vi "Romi-Robot-Simulation.vi"() -> ()   [LabVIEW 2019]
doc: "This WebSockets API example VI acts as a server for an incoming websockets connection. Receives/sends string data to the connected client."
uses:
  <vilib>/Rock Robotics/WPI/Simulation/Protocol/Devices/RoboRIO/RoboRIO Update Ops.ctl
  <vilib>/Rock Robotics/WPI/Simulation/Protocol/Devices/DriverStation/DS Update Ops.ctl
  <vilib>/Rock Robotics/WPI/Simulation/Protocol/Devices/DIO/DIO Update Ops.ctl
  <vilib>/Rock Robotics/SystemInterfaces/DIO/FPGA_DIOChannel.ctl
  <vilib>/Utility/miscctls.llb/LVBoundsTypeDef.ctl
  <vilib>/Rock Robotics/WPI/ThirdParty/JAS_Junk/TrajLib/Trajectory_Library.lvlib
  <vilib>/mediamongrels ltd/websockets/websockets/websocket server/WebSocket Server.lvclass
  C:/Program Files (x86)/National Instruments/LabVIEW 2020/vi.lib/mediamongrels ltd/websockets/websockets/websocket/WebSocket.lvclass
  <vilib>/Rock Robotics/WPI/Simulation/Protocol/Devices/PWM/PWM data proto.ctl
  <vilib>/Rock Robotics/WPI/Simulation/Protocol/Devices/PWM/PWM proto.ctl
  <vilib>/Rock Robotics/WPI/Simulation/Protocol/Devices/RoboRIO/RoboRIO data proto.ctl
  <vilib>/Rock Robotics/WPI/Simulation/Protocol/Devices/RoboRIO/RoboRIO proto.ctl
  <vilib>/Rock Robotics/WPI/Simulation/Protocol/Devices/DriverStation/DS data proto.ctl
  <vilib>/Rock Robotics/WPI/Simulation/Protocol/Devices/DriverStation/DS proto.ctl
  <vilib>/Rock Robotics/WPI/Simulation/Protocol/Devices/DIO/DIO data proto.ctl
  <vilib>/Rock Robotics/WPI/Simulation/Protocol/Devices/DIO/DIO proto.ctl
  <vilib>/Rock Robotics/WPI/Simulation/Protocol/Devices/Encoder/Encoder data protoo.ctl
  <vilib>/Rock Robotics/WPI/Simulation/Protocol/Devices/Encoder/Encoder proto.ctl
  <vilib>/Analysis/Matrix/Datatypes/RealMatrix.ctl
  <vilib>/Analysis/Matrix/NI_Matrix.lvlib
  <vilib>/Rock Robotics/WPI/ThirdParty/JAS_Junk/TrajLib/TypeDef/LINEAR_SYSTEM.ctl
  <vilib>/Rock Robotics/WPI/ThirdParty/JAS_Junk/TrajLib/TypeDef/DCMOTOR.CTL
  <vilib>/Rock Robotics/WPI/ThirdParty/JAS_Junk/TrajLib/TypeDef/DIFF_DRIVE_TRAIN_SIM.ctl
  <vilib>/vision/Image Controls.llb/IMAQ Image.ctl
  ROBOT_PICTURE.ctl
  <vilib>/Rock Robotics/WPI/Simulation/Protocol/Devices/Gyro/Gyro Data proto.ctl
  <vilib>/Rock Robotics/WPI/Simulation/Protocol/Devices/Gyro/Gyro proto.ctl
panel:
  in  "Tab Control":T1(tab)
  in  "Start Simulation":bool
  in  "Field Selector":string(combo)
  in  "Robot Y Position\nInches":dbl=84.0
  in  "Robot X Position\nInches":dbl=120.0
  in  "Robot Orientation\nDegrees":dbl
  out "Heading Deg":dbl format="%11.1f"
  out "Right Wheel\nInch / Sec":dbl format="%11.1f"
  out "Left Wheel\nInch / Sec":dbl format="%11.1f"
  in  "Button\n    C":bool
  in  "Button\n    B":bool
  out "Yellow LED\nDIO 3":bool
  out "Green LED\nDIO 1":bool
  out "Red LED\nDIO 2":bool
  in  "Button\n    A":bool
  out "RSL ON":picture
  out "ROBOT":T2
  out "RSL OFF":picture
  out "Field Picture":picture
  out "Y Pos Inch":dbl format="%11.1f"
  out "X Pos Inch":dbl format="%11.1f"
  out "Gyro":T3={"type"="Gyro", "device"="", "name"="", "data"={"<init"=0, ">connected"=FALSE, "<offsetX"=0.0, "<offsetY"=0.0, "<offsetZ"=0.0, ">angle_x"=0.0, ">angle_y"=0.0, ">angle_z"=0.0, ">rate_x"=0.0, ">rate_y"=0.0, ">rate_z"=0.0, "<gain"=0.0}}
  out "DIO 0\nIn":T5={"type"="DIO", "device"="", "name"="", "data"={"<init"=FALSE, "<>value"=FALSE, "<pulse_length"=0, "<input"=FALSE}}
  out "Enc Left":T7={"type"="Encoder", "device"="", "name"="", "data"={"<init"=FALSE, ">count"=0.0, ">period"=0.0, "<samples_to_avg"=0, "<offset"=0.0, "<channel_a"=0, "<channel_b"=0}}
  out "Enc Right":T7={"type"="Encoder", "device"="", "name"="", "data"={"<init"=FALSE, ">count"=0.0, ">period"=0.0, "<samples_to_avg"=0, "<offset"=0.0, "<channel_a"=0, "<channel_b"=0}}
  out "DIO 1\nIn / Out":T5={"type"="DIO", "device"="", "name"="", "data"={"<init"=FALSE, "<>value"=FALSE, "<pulse_length"=0, "<input"=FALSE}}
  out "DIO 2\nIn / Out":T5={"type"="DIO", "device"="", "name"="", "data"={"<init"=FALSE, "<>value"=FALSE, "<pulse_length"=0, "<input"=FALSE}}
  out "PWM 0":T9
  out "PWM 1":T9
  out "DIO 3\nOut":T5={"type"="DIO", "device"="", "name"="", "data"={"<init"=FALSE, "<>value"=FALSE, "<pulse_length"=0, "<input"=FALSE}}
  out "roboRIO":T11={"type"="roboRIO", "device"="", "name"="", "data"={">fpga_button"=FALSE, ">vin_voltage"=0.0, ">vin_current"=0.0, ">6v_voltage"=0.0, ">6v_current"=0.0, ">6v_active"=FALSE, ">6v_faults"=0.0, ">5v_voltage"=0.0, ">5v_current"=0.0, ">5v_active"=FALSE, ">5v_faults"=0.0, ">3v3_voltage"=0.0, ">3v3_current"=0.0, ">3v3_active"=FALSE, ">3v3_faults"=0.0}}
  out "Driverstation":T13={"type"="Driverstation", "device"="", "name"="", "data"={">enabled"=FALSE, ">autonomous"=FALSE, ">test"=FALSE, ">estop"=FALSE, ">fms"=FALSE, ">ds"=FALSE, "<match_time"=0.0, ">station"="", ">game_data"=""}}
  out "Request URI":string
  out "HTTP Headers":variant
  out "Stop Sim":bool
  out "Battery Voltage VDC":dbl format="%18.2f"
  out "Gyro Reading   Deg":dbl format="%19.3f"
  out "Edges/Feet":dbl
  out "out DiffDriveTrainSim":T15 {"m_Motor"."Jr_KgM2" format="%13.5p"; "m_Motor"."L_H" format="%13.5p"; "m_Motor"."Kt_NMPerAmp" format="%13.5p"; "m_Motor"."KvINV_RadPerSecPerVolt" format="%13.5p"; "m_Motor"."R_Ohms" format="%13.5p"; "m_Motor"."FreeSpeed_RadPerSec" format="%13.5p"; "m_Motor"."FreeCurrent_Amps" format="%13.5p"; "m_Motor"."StallCurrent_Amps" format="%13.5p"; "m_Motor"."StallTorque_NM" format="%13.5p"; "m_Motor"."nominalVoltage_Volts" format="%13.5p"}
  out "Speed Left  Ft/Sec":dbl format="%13.2f"
  out "Speed Right  Ft/Sec":dbl format="%13.2f"
  out "Amps":dbl
  out "PWM 0 Rate":dbl format="%19.3f"
  out "PWM 1 Rate":dbl format="%19.3f"
  out "FIeld Image":T19
  out "Y Pos Pixel":dbl format="%11.1f"
  out "X Pos Pixel":dbl format="%11.1f"
  # "Romi Switches/Lights"
  # "Robot Position"
  # "Robot Speed"
  # "Dig In 0"
  # "Dig In 1"
  # "Dig In 2"
  # "<States, 1>"
  # "<Outputs, 1>"
  # "<Inputs, 1>"
  # "<Outputs, 1>"
  # "<States,States>"
  # "<States,Inputs>"
  # "<Outputs,States>"
  # "<Outputs,Inputs>"
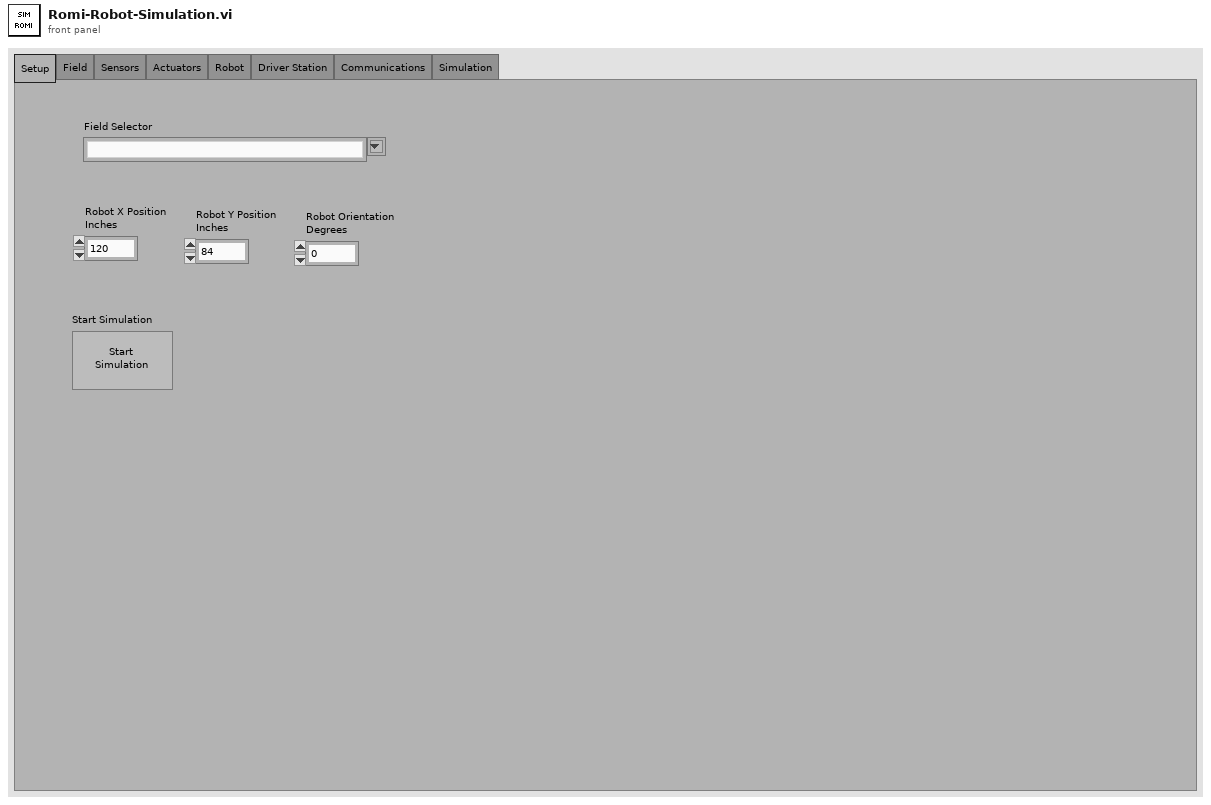
[diagram p1: front panel]
types:
  T1 = enum32{"Setup", "Field", "Sensors", "Actuators", "Robot", "Driver Station", "Communications", "Simulation"}
  T2 = typedef "ROBOT_PICTURE.ctl" = picture
  T3 = typedef "Gyro proto.ctl" = cluster{"type":string, "device":string, "name":string, "data":T4}
  T4 = typedef "Gyro Data proto.ctl" = cluster{"<init":i32, ">connected":bool, "<offsetX":dbl, "<offsetY":dbl, "<offsetZ":dbl, ">angle_x":dbl, ">angle_y":dbl, ">angle_z":dbl, ">rate_x":dbl, ">rate_y":dbl, ">rate_z":dbl, "<gain":dbl}
  T5 = typedef "DIO proto.ctl" = cluster{"type":string, "device":string, "name":string, "data":T6}
  T6 = typedef "DIO data proto.ctl" = cluster{"<init":bool, "<>value":bool, "<pulse_length":i32, "<input":bool}
  T7 = typedef "Encoder proto.ctl" = cluster{"type":string, "device":string, "name":string, "data":T8}
  T8 = typedef "Encoder data protoo.ctl" = cluster{"<init":bool, ">count":dbl, ">period":dbl, "<samples_to_avg":i32, "<offset":dbl, "<channel_a":i32, "<channel_b":i32}
  T9 = typedef "PWM proto.ctl" = cluster{"type":string, "device":string, "name":string, "data":T10}
  T10 = typedef "PWM data proto.ctl" = cluster{"<init":bool, "<speed":dbl, "<position":dbl, "<raw":dbl, "<period_scale":dbl, "<zero_latch":bool, "<servo range":dbl}
  T11 = typedef "RoboRIO proto.ctl" = cluster{"type":string, "device":string, "name":string, "data":T12}
  T12 = typedef "RoboRIO data proto.ctl" = cluster{">fpga_button":bool, ">vin_voltage":dbl, ">vin_current":dbl, ">6v_voltage":dbl, ">6v_current":dbl, ">6v_active":bool, ">6v_faults":dbl, ">5v_voltage":dbl, ">5v_current":dbl, ">5v_active":bool, ">5v_faults":dbl, ">3v3_voltage":dbl, ">3v3_current":dbl, ">3v3_active":bool, ">3v3_faults":dbl}
  T13 = typedef "DS proto.ctl" = cluster{"type":string, "device":string, "name":string, "data":T14}
  T14 = typedef "DS data proto.ctl" = cluster{">enabled":bool, ">autonomous":bool, ">test":bool, ">estop":bool, ">fms":bool, ">ds":bool, "<match_time":dbl, ">station":string, ">game_data":string}
  T15 = typedef "Trajectory_Library.lvlib/DIFF_DRIVE_TRAIN_SIM.ctl" = cluster{"m_Plant":T16, "m_X":T17, "m_Y":T17, "m_U":T17, "MeasureStdDev":T17, "m_Motor":T18, "m_OriginalGearing":dbl, "m_CurrentGearing":dbl, "m_WheelRadius_M":dbl, "m_RB":dbl}
  T16 = typedef "Trajectory_Library.lvlib/LINEAR_SYSTEM.ctl" = cluster{"m_A":T17, "m_B":T17, "m_C":T17, "m_D":T17, "States":i32, "Inputs":i32, "Outputs":i32}
  T17 = typedef "NI_Matrix.lvlib/RealMatrix.ctl" = dbl[][]
  T18 = typedef "Trajectory_Library.lvlib/DCMOTOR.CTL" = cluster{"nominalVoltage_Volts":dbl, "StallTorque_NM":dbl, "StallCurrent_Amps":dbl, "FreeCurrent_Amps":dbl, "FreeSpeed_RadPerSec":dbl, "R_Ohms":dbl, "KvINV_RadPerSecPerVolt":dbl, "Kt_NMPerAmp":dbl, "L_H":dbl, "Jr_KgM2":dbl}
  T19 = typedef "IMAQ Image.ctl" = refnum<image>
  T20 = typedef "LVBoundsTypeDef.ctl" = cluster{"Width":u32, "Height":u32}
  T21 = typedef "Image Type" = u32
  T22 = typedef "TrajectoryUtils_Field_Info.ctl" = cluster{"FIeld_File_Name":string, "Top_Left_X":i32, "Top_Left_Y":i32, "Bottom_Right_X":i32, "Bottom_Right_Y":i32, "Field_Size_X":dbl, "Field_Size_Y":dbl, "FIeld_Size_Units":string}
  T23 = typedef "Trajectory_Library.lvlib/POSE2D.ctl" = cluster{"TRANSLATION":T24, "ROTATION":T25}
  T24 = typedef "Trajectory_Library.lvlib/TRANSLATION2D.ctl" = cluster{"X":dbl, "Y":dbl}
  T25 = typedef "Trajectory_Library.lvlib/ROTATION2D.ctl" = cluster{"VALUE":dbl, "COS":dbl, "SIN":dbl}
  T26 = typedef "Rotated_Picture_TypeDef.ctl" = cluster{"ONE-8-bit pixmap":u8[][], "Two-Array":cdb[][], "Three-Numeric":i32, "Four-Numeric":i32, "Five-Numeric":cdb, "Six-colors":u32[], "Seven-new element/subarray":u32, "Eight-Cluster":cluster{"[0]":i32, "[1]":i32}}
  T27 = typedef "FPGA_DIOChannel.ctl" = enum8{"DIO 0", "DIO 1", "DIO 2", "DIO 3", "DIO 4", "DIO 5", "DIO 6", "DIO 7", "DIO 8", "DIO 9", "DIO MXP 0", "DIO MXP 1", "DIO MXP 2", "DIO MXP 3", "DIO MXP 4", "DIO MXP 5", "DIO MXP 6", "DIO MXP 7", "DIO MXP 8", "DIO MXP 9", "DIO MXP 10", "DIO MXP 11", "DIO MXP 12", "DIO MXP 13", "DIO MXP 14", "DIO MXP 15", "SPI Port CS1", "SPI Port CS2", "SPI Port CS3", "SPI Port MISO", "SPI Port MOSI", "Invalid"}
  T28 = typedef "DIO Update Ops.ctl" = enum16{"set init", "set value", "set pulse_length", "set input", "get", "delete", "JSON update", "set name", "transmit initial", "reset"}
  T29 = typedef "DS Update Ops.ctl" = enum16{"set enabled", "set autonomous", "set test", "set estop", "set fms", "set ds", "set control word", "set match_time", "set station", "set game data", "JSON update", "set name", "get", "transmit initial", "reset"}
  T30 = typedef "RoboRIO Update Ops.ctl" = enum16{"get", "JSON update", "set name", "transmit initial", "set fpga_button", "set vin_voltage", "set vin_current", "set 6v_voltage", "set 6v_current", "set 6v_active", "set 6v_faults", "set 5v_voltage", "set 5v_current", "set 5v_active", "set 5v_faults", "set 3v3_voltage", "set 3v3_current", "set 3v3_active", "set 3v3_faults", "reset"}
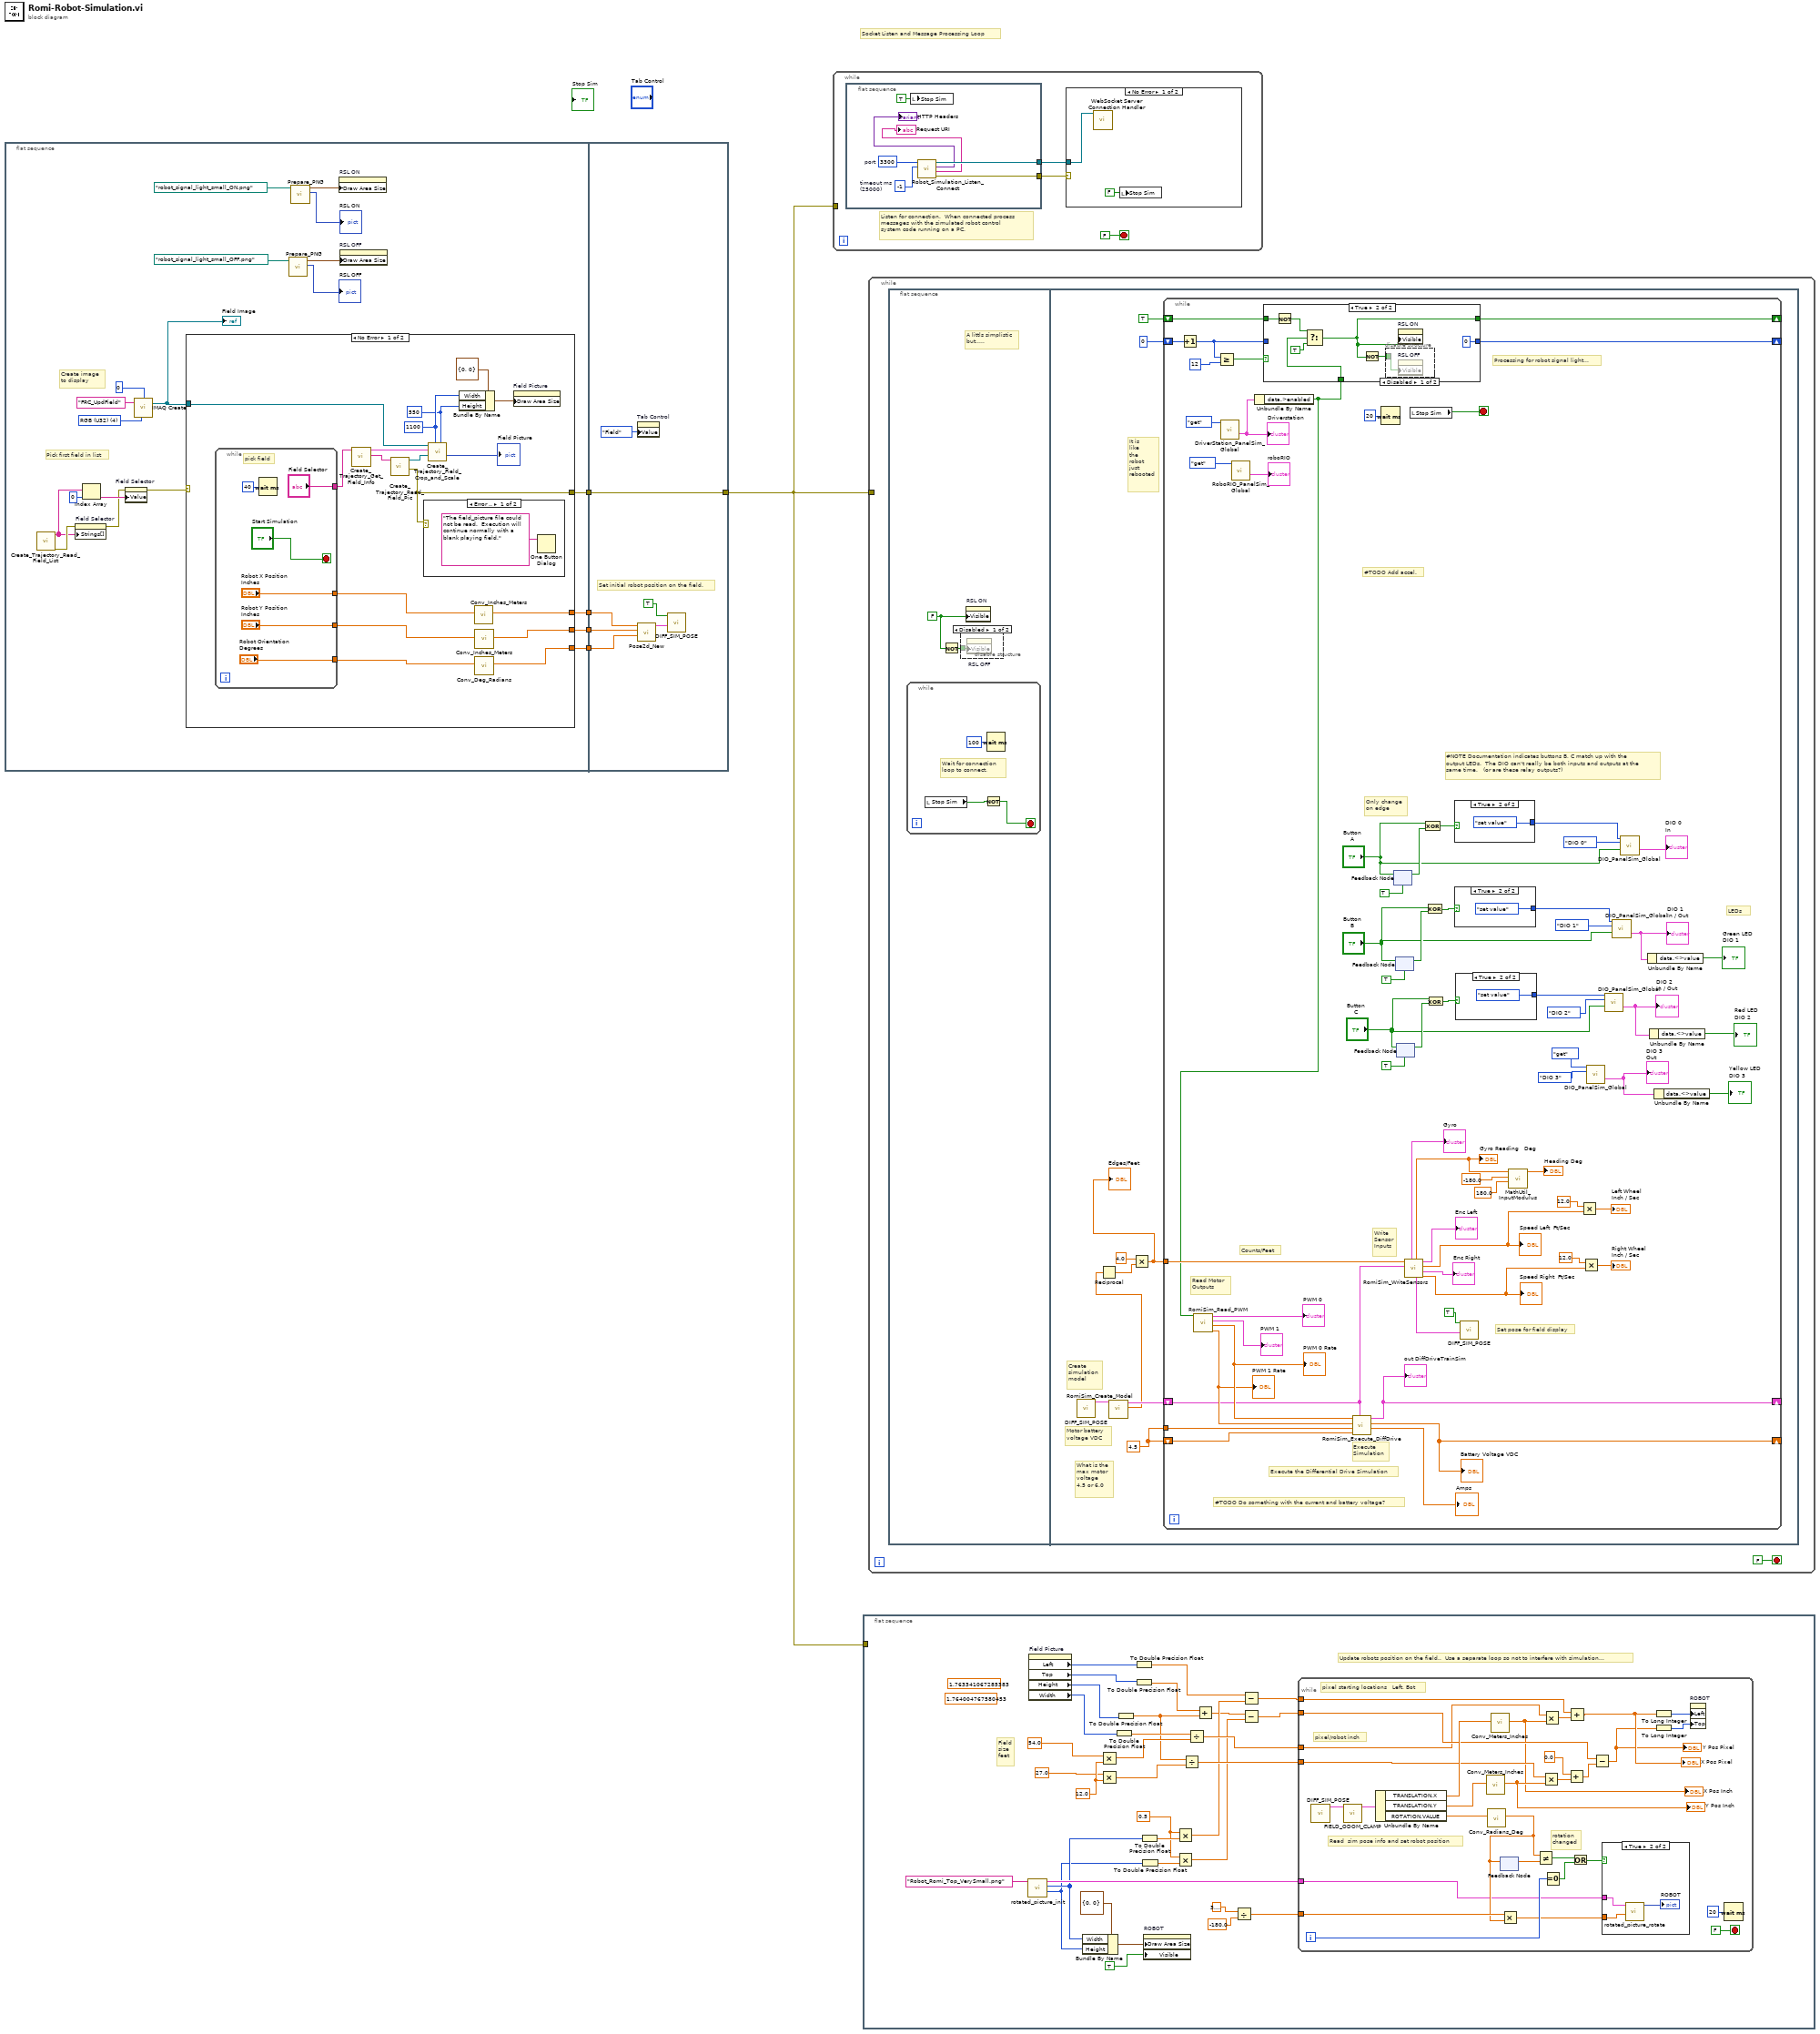
[diagram p0: block diagram]
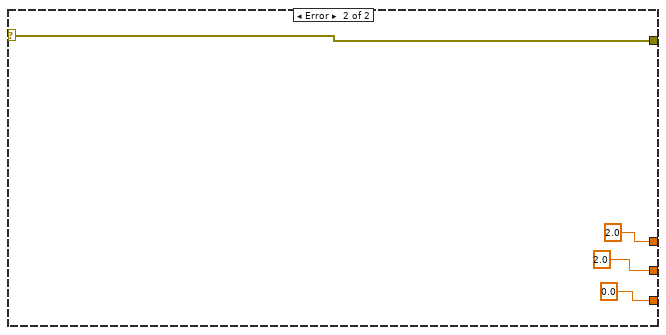
[diagram p4: hidden frame]
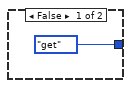
[diagram p6: hidden frame]
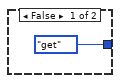
[diagram p7: hidden frame]
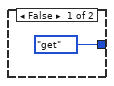
[diagram p8: hidden frame]
diagram:
  # "Socket Listen and Message Processing Loop"
  n1 = flat-sequence {
    tunnel: [w18] -> w5
    tunnel: [w8] -> w3
    tunnel: [w7] -> w2
    tunnel: [w6] -> w1
    tunnel: [w60] -> w4
    tunnel: w5 -> [w60]
    tunnel: w3 -> [w56]
    tunnel: w2 -> [w55]
    tunnel: w1 -> [w54]
    frame #0 {
      w23 = T21 4 items=["Grayscale (U8)", "Grayscale (I16)", "Grayscale (SGL)", "Complex (CSG)", "RGB (U32)", "HSL (U32)", "RGB (U64)", "Grayscale (U16)"] ("Image Type")
      # "Pick first field in list"
      # "Create image \nto display"
      n2 = call "Create_Trajectory_Read_Field_List.vi"() -> ("error out"=w14:errorcluster, "section names"=w13:string[])  [unwired: 10 in]
      n3 = property on="Field Selector" class="CmbBox"(error in=w14, "Strings[]"=w13) -> (error out=w10:errorcluster)  [unwired: 1 in, 1 out]
      n4 = Index Array(array=w13, index=0) -> (element=w11:string)
      n5 = property on="Field Selector" class="CmbBox"(error in=w10, "Value"=w11) -> (error out=w9:errorcluster)  [unwired: 1 in, 1 out]
      n6 = call "IMAQ Create"("Border Size"=0, "Image Name"="FRC_UpdField", "Image Type"=w23) -> ("New Image"=w22:T19)  [unwired: 2 in, 1 out]
      "FIeld Image" <- w22
      n7 = case shown="No Error" w9 {
        selector: w9 -> [_ w53]
        tunnel: w22 -> [w33 _]
        tunnel: [w39 w53] -> w18
        tunnel: [w28 2.0 ("Meters")] -> w8
        tunnel: [w27 2.0 ("Meters")] -> w7
        tunnel: [w26 0.0 ("Radians")] -> w6
        frame No Error {
          w34 = 550 ("Disp Y Size Pixel")
          w35 = 1100 ("Disp X Size Pixel")
          n8 = while {
            tunnel: ["Field Selector"] -> w32
            tunnel: ["Robot X Position\nInches"] -> w31
            tunnel: ["Robot Y Position\nInches"] -> w30
            tunnel: ["Robot Orientation\nDegrees"] -> w29
            stop <- "Start Simulation" stop-if-true
            # "pick field"
            n9 = Wait (ms)(milliseconds to wait=u32 40) -> ()  [unwired: 1 out]
          }
          n10 = call "Create_Trajectory_Get_Field_Info.vi"("Field Selector"=w32) -> ("File"=w42:string, "input cluster"=w41:T22)  [unwired: 9 in]
          n11 = call "Create_Trajectory_Read_Field_Pic.vi"("file name"=w42) -> ("Image Error"=w39:errorcluster, "Image Data"=w40:T19)  [unwired: 7 in, 2 out]
          n12 = case shown="Error .." w39 {
            frame Error {
              n13 = One Button Dialog(message="The field_picture file could not be read.  Execution will continue normally with a blank playing field.") -> ()  [unwired: 1 in, 1 out]
            }
            frame No Error {
            }
          }
          n14 = call "Create_Trajectory_Field_Crop_and_Scale.vi"("Disp Y Size Pixel"=w34, "Disp X Size Pixel"=w35, "Field Image"=w40, "field Info"=w41, "Display Image"=w33) -> ("Cropped Field Picture Out"=→"Field Picture":picture)  [unwired: 4 in, 2 out]
          n15 = Bundle By Name(cluster=T20 {"Width"=0, "Height"=0} ("Draw Area Size"), "Width"=w35, "Height"=w34) -> (w36:T20)
          n16 = call <vilib>:"Conv_Inches_Meters.vi"("INCH"=w31) -> ("Meters"=w28:dbl)  [unwired: 10 in]
          n17 = call <vilib>:"Conv_Inches_Meters.vi"("INCH"=w30) -> ("Meters"=w27:dbl)  [unwired: 10 in]
          n18 = call <vilib>:"Conv_Deg_Radians.vi"("Degress"=w29) -> ("Radians"=w26:dbl)  [unwired: 10 in]
          n19 = property on="Field Picture" class="Pict"("Draw Area Size"=w36) -> ()  [unwired: 2 in, 2 out]
        }
        frame Error {
        }
      }
      n20 = call "Prepare_PNG.vi"("path to PNG file"=path "robot_signal_light_small_OFF.png") -> ("new picture"=→"RSL OFF":picture, "Draw Area Size"=w17:T20)  [unwired: 9 in]
      n21 = call "Prepare_PNG.vi"("path to PNG file"=path "robot_signal_light_small_ON.png") -> ("new picture"=→"RSL ON":picture, "Draw Area Size"=w20:T20)  [unwired: 9 in]
      n22 = property on="RSL ON" class="Pict"("Draw Area Size"=w20) -> ()  [unwired: 2 in, 2 out]
      n23 = property on="RSL OFF" class="Pict"("Draw Area Size"=w17) -> ()  [unwired: 2 in, 2 out]
    }
    frame #1 {
      # "Set initial robot position on the field."
      n24 = property on="Tab Control" class="TabCtl (strict)"("Value"=T1."Field" ("Tab Control")) -> ()  [unwired: 2 in, 2 out]
      n25 = call <vilib>:"Pose2d_New.vi"("Heading"=w54, "Y"=w55, "X"=w56) -> ("out POSe"=w59:T23)  [unwired: 8 in]
      n26 = call "DIFF_SIM_POSE.vi"("in Sim Pose"=w59, "WRITE"=TRUE) -> ()  [unwired: 9 in, 1 out]
    }
  }
  n27 = while {
    tunnel: w4 -> [_]
    stop <- FALSE stop-if-true
    # "Listen for connection.  When connected process\nmessages with the simulated robot control\nsystem code running on a PC."
    n28 = flat-sequence {
      tunnel: [w68] -> w62
      tunnel: [w66] -> w61
      frame #0 {
        w69 = -1  # timeout ms  (25000)
        w70 = u16 3300  # port
        n29 = local write "Stop Sim"(TRUE ("Stop\nSim")) -> ()
        n30 = call <vilib>:"Robot_Simulation_Listen_Connect.vi"("timeout ms (25000)"=w69, "port"=w70) -> ("error out"=w68:errorcluster, "Properties:Request URI"=→"Request URI":string, "Properties:Return Headers"=→"HTTP Headers":variant, "WebSocket Connection out"=w66:refnum<class "WebSocket Server.lvclass">)  [unwired: 6 in]
      }
    }
    n31 = case shown="No Error" w62 {
      tunnel: w61 -> [w71 _]
      frame No Error {
        n32 = call <vilib>:"WebSocket Server Connection Handler.vi"("WebSocket in"=w71) -> ()  [unwired: 10 in, 1 out]
        n33 = local write "Stop Sim"(FALSE ("Stop\nSim")) -> ()
      }
      frame Error {
      }
    }
  }
  n34 = flat-sequence {
    tunnel: w4 -> [_]
    frame #0 {
      w82 = 0.5
      (unwired) 1.764004767580453
      (unwired) 1.763341067285383
      w100 = 12.0 ("y")
      # "Field\nsize\nfeet"
      # "Update robots position on the field..  Use a separate loop so not to interfere with simulation..."
      n35 = call "rotated_picture_init.vi"("Picture FIle Name"="Robot_Romi_Top_VerySmall.png" ("name or relative path")) -> ("Height"=w74:i16, "Width"=w75:i16, "RotatedPictureInfo"=w101:T26)  [unwired: 7 in, 1 out]
      n36 = property on="Field Picture" class="Pict"() -> ("Left"=w97:i32, "Top"=w96:i32, "Height"=w95:u32, "Width"=w94:u32)  [unwired: 2 in, 2 out]
      n37 = Bundle By Name(cluster=T20 {"Width"=0, "Height"=0} ("Draw Area Size"), "Width"=w75, "Height"=w74) -> (w77:T20)
      n38 = Multiply(x=54.0, y=w100) -> (x*y=w91:dbl)
      n39 = Multiply(x=27.0, y=w100) -> (x*y=w88:dbl)
      n40 = To Double Precision Float(number=w94) -> (double precision float=w92:dbl)
      n41 = To Double Precision Float(number=w95) -> (double precision float=w89:dbl)
      n42 = To Double Precision Float(number=w97) -> (double precision float=w81:dbl)
      n43 = To Double Precision Float(number=w96) -> (double precision float=w93:dbl)
      n44 = To Double Precision Float(number=w75) -> (double precision float=w84:dbl)
      n45 = To Double Precision Float(number=w74) -> (double precision float=w83:dbl)
      n46 = property on="ROBOT" class="Pict (strict)"("Draw Area Size"=w77, "Visible"=TRUE) -> ()  [unwired: 2 in, 2 out]
      n47 = Multiply(x=w82, y=w84) -> (x*y=w80:dbl)
      n48 = Multiply(x=w82, y=w83) -> (x*y=w78:dbl)
      n49 = Divide(x=w89, y=w88) -> (x/y=w87:dbl)
      n50 = Divide(x=w92, y=w91) -> (x/y=w90:dbl)
      n51 = Add(x=w93, y=w89) -> (x+y=w79:dbl)
      n52 = Divide(x=3.141592653589793, y=-180.0 ("value")) -> (x/y=w105:dbl)
      n53 = Subtract(x=w81, y=w80) -> (x-y=w86:dbl)
      n54 = Subtract(x=w79, y=w78) -> (x-y=w85:dbl)
      n55 = while {
        tunnel: w105 -> [w135]
        tunnel: w101 -> [w118]
        tunnel: w86 -> [w115]
        tunnel: w85 -> [w114]
        tunnel: w90 -> [w113]
        tunnel: w87 -> [w112]
        i -> [w124]
        stop <- FALSE stop-if-true
        # "pixel starting locations   Left, Bot"
        # "Read  sim pose info and set robot position"
        # "pixel/robot inch"
        # "rotation\nchanged"
        n56 = call "DIFF_SIM_POSE.vi"() -> ("out Sim Pose"=w117:T23)  [unwired: 11 in]
        n57 = call "FIELD_ODOM_CLAMP.vi"("in Sim Pose"=w117) -> ("out Sim Pose"=w116:T23)  [unwired: 10 in]
        n58 = Unbundle By Name(w116) -> ("TRANSLATION.X"=w123:dbl, "TRANSLATION.Y"=w122:dbl, "ROTATION.VALUE"=w120:dbl)
        n59 = call <vilib>:"Conv_Meters_Inches.vi"("Meters"=w122) -> ("Inches"=w107:dbl)  [unwired: 10 in]
        "Y Pos Inch" <- w107
        n60 = call <vilib>:"Conv_Radians_Deg.vi"("Radians"=w120) -> ("Degrees"=w121:dbl)  [unwired: 10 in]
        n61 = call <vilib>:"Conv_Meters_Inches.vi"("Meters"=w123) -> ("Inches"=w106:dbl)  [unwired: 10 in]
        "X Pos Inch" <- w106
        n62 = feedback-in #1(w121) -> ()
        n63 = feedback #1() -> (w132:dbl)  [unwired: 1 in]
        n64 = Multiply(x=w135, y=w121) -> (x*y=w119:dbl)
        n65 = Not Equal?(x=w121, y=w132) -> (x != y?=w126:bool)
        n66 = Multiply(x=w112, y=w107) -> (x*y=w130:dbl)
        n67 = Multiply(x=w113, y=w106) -> (x*y=w131:dbl)
        n68 = Equal To 0?(x=w124) -> (x = 0?=w125:bool)
        n69 = Add(x=0.0, y=w130) -> (x+y=w128:dbl)
        n70 = Add(x=w115, y=w131) -> (x+y=w109:dbl)
        "X Pos Pixel" <- w109
        n71 = Or(x=w126, y=w125) -> (x .or. y?=w127:bool)
        n72 = Subtract(x=w114, y=w128) -> (x-y=w108:dbl)
        "Y Pos Pixel" <- w108
        n73 = case shown="True" w127 {
          tunnel: w119 -> [_ w136]
          tunnel: w118 -> [_ w137]
          frame False {
          }
          frame True {
            n74 = call "rotated_picture_rotate.vi"("Angle"=w136, "RotatedPictureInfo"=w137) -> ("new picture"=→"ROBOT":picture)  [unwired: 9 in]
          }
        }
        n75 = To Long Integer(number=w109) -> (32bit integer=w111:i32)
        n76 = To Long Integer(number=w108) -> (32bit integer=w110:i32)
        n77 = property on="ROBOT" class="Pict (strict)"("Left"=w111, "Top"=w110) -> ()  [unwired: 2 in, 2 out]
        n78 = Wait (ms)(milliseconds to wait=u32 20) -> ()  [unwired: 1 out]
      }
    }
  }
  n79 = while {
    tunnel: w4 -> [_]
    stop <- FALSE stop-if-true
    n80 = flat-sequence {
      frame #0 {
        w140 = FALSE ("Visible")
        # "A littls simplistic\nbut....."
        n81 = while {
          stop <- w143 stop-if-true
          # "Wait for connection\nloop to connect."
          n82 = local read "Stop Sim"() -> (w144:bool)
          n83 = Not(x=w144) -> (.not. x?=w143:bool)
          n84 = Wait (ms)(milliseconds to wait=u32 100) -> ()  [unwired: 1 out]
        }
        n85 = Not(x=w140) -> (.not. x?=w141:bool)
        n86 = disable-structure shown="Disabled" {
          disable-tunnel: w141 -> [w142 _]
          frame Disabled {
            n87 = property on="RSL OFF" class="Pict"("Visible"=w142) -> ()  [unwired: 2 in, 2 out]
          }
          frame Enabled {
          }
        }
        n88 = property on="RSL ON" class="Pict"("Visible"=w140) -> ()  [unwired: 2 in, 2 out]
      }
      frame #1 {
        w147 = 4.5 ("Voltage")
        # "Create\nsimulation\nmodel"
        # "Motor battery\nvoltage VDC"
        # "What is the\nmax motor\nvoltage\n4.5 or 6.0"
        # "It is\nlike\nthe \nrobot \njust\nrebooted"
        n89 = call "DIFF_SIM_POSE.vi"() -> ("out Sim Pose"=w146:T23)  [unwired: 11 in]
        n90 = call "RomiSim_Create_Model.vi"("Initial Robot Position"=w146) -> ("Encoder Ft/Count"=w149:dbl, "out DiffDriveTrainSim"=w152:T15)  [unwired: 9 in]
        n91 = Reciprocal(x=w149) -> (1/x=w150:dbl)
        n92 = Multiply(x=4.0, y=w150) -> (x*y=w148:dbl)
        "Edges/Feet" <- w148
        n93 = while {
          shift-right: [w205] -> _
          shift-left: 0 -> [w210]
          shift-right: [w207] -> _
          shift-left: TRUE -> [w208]
          shift-right: [w201] -> _
          shift-left: w152 -> [w170]
          shift-right: [w200] -> _
          shift-left: w147 -> [w168]
          tunnel: w148 -> [w199]
          tunnel: w147 -> [w169]
          stop <- w212 stop-if-true
          # "Execute\nSimulation"
          # "Write\nSensor\nInputs"
          # "Read Motor\nOutputs"
          # "Only change\non edge"
          # "LEDs"
          # "#NOTE Documentation indicates buttons B, C match up with the\noutput LEDs.  The DIO can't really be both inputs and outputs at the\nsame time.   (or are these relay outputs?)"
          # "#TODO Add accel."
          # "#TODO Do something with the current and battery voltage?"
          # "Counts/Feet"
          # "Set pose for field display"
          # "Execute the Differential Drive Simulation"
          # "Processing for robot signal light..."
          n94 = Increment(x=w210) -> (x+1=w206:i32)
          n95 = Greater Or Equal?(x=w206, y=12) -> (x >= y?=w204:bool)
          n96 = call <vilib>:"DriverStation_PanelSim_Global.vi"("menu"=DS_Update_Ops."get") -> ("Driverstation new"=w211:T13)  [unwired: 13 in, 1 out]
          "Driverstation" <- w211
          n97 = call <vilib>:"RoboRIO_PanelSim_Global.vi"("Menu"=RoboRIO_Update_Ops."get") -> ("roboRIO new"=→"roboRIO":T11)  [unwired: 13 in, 1 out]
          n98 = Unbundle By Name(w211) -> ("data.>enabled"=w197:bool)
          n99 = call "RomiSim_Read_PWM.vi"("Robot Enabled"=w197) -> ("Right Motor Dmd"=w171:dbl, "Left Motor Dmd"=w198:dbl, "Right PWM Sim"=→"PWM 1":T9, "Left PWM Sim"=→"PWM 0":T9)  [unwired: 7 in]
          "PWM 0 Rate" <- w198
          "PWM 1 Rate" <- w171
          n100 = case shown="True" w204 {
            tunnel: w208 -> [w229 w236]
            tunnel: [w229 w231] -> w207
            tunnel: w206 -> [w228 _]
            tunnel: [w228 0] -> w205
            tunnel: w197 -> [_ w234]
            frame False {
            }
            frame True {
              n101 = Not(x=w236) -> (.not. x?=w235:bool)
              n102 = Select(t=w235, s=w234, f=TRUE) -> (s? t:f=w231:bool)
              n103 = Not(x=w231) -> (.not. x?=w232:bool)
              n104 = disable-structure shown="Disabled" {
                disable-tunnel: w232 -> [w237 _]
                frame Disabled {
                  n105 = property on="RSL OFF" class="Pict"("Visible"=w237) -> ()  [unwired: 2 in, 2 out]
                }
                frame Enabled {
                }
              }
              n106 = property on="RSL ON" class="Pict"("Visible"=w231) -> ()  [unwired: 2 in, 2 out]
            }
          }
          n107 = call "RomiSim_Execute_DiffDrive.vi"("out DiffDriveTrainSim in"=w170, "Actual  Battery Voltage"=w168, "Nominal Battery Voltage"=w169, "Right Motor Dmd"=w171, "Left Motor Dmd"=w198) -> ("Current Amps"=→"Amps":dbl, "Battery Volts"=w200:dbl, "out DiffDriveTrainSim out"=w201:T15)  [unwired: 4 in]
          "out DiffDriveTrainSim" <- w201
          "Battery Voltage VDC" <- w200
          n108 = Wait (ms)(milliseconds to wait=u32 20) -> ()  [unwired: 1 out]
          n109 = feedback-in #2("Button\n    A") -> ()
          n110 = feedback #2(TRUE) -> (w194:bool)
          n111 = feedback #3(TRUE) -> (w191:bool)
          n112 = feedback-in #3("Button\n    B") -> ()
          n113 = feedback #4(TRUE) -> (w188:bool)
          n114 = feedback-in #4("Button\n    C") -> ()
          n115 = call "RomiSim_WriteSensors.vi"("Diff Drive Train Sim"=w170, "Counts/Feet"=w199) -> ("Right Speed Ft/Sec"=w160:dbl, "Right Encoder"=→"Enc Right":T7, "Left Speed Ft/Sec"=w163:dbl, "Left Encoder"=→"Enc Left":T7, "Robot Pose"=w167:T23, "Gyro Deg"=w158:dbl, "Gyro"=→"Gyro":T3)  [unwired: 3 in]
          "Gyro Reading   Deg" <- w158
          "Speed Right  Ft/Sec" <- w160
          "Speed Left  Ft/Sec" <- w163
          n116 = local read "Stop Sim"() -> (w212:bool)
          n117 = Exclusive Or(1:w194, 2:"Button\n    A") -> (0:w193:bool)
          n118 = Exclusive Or(1:w191, 2:"Button\n    B") -> (0:w190:bool)
          n119 = Exclusive Or(1:w188, 2:"Button\n    C") -> (0:w187:bool)
          n120 = case shown="True" w193 {
            tunnel: [DIO_Update_Ops."get" ("menu") DIO_Update_Ops."set value" ("menu")] -> w175
            frame False {
            }
            frame True {
            }
          }
          n121 = case shown="True" w190 {
            tunnel: [DIO_Update_Ops."get" ("menu") DIO_Update_Ops."set value" ("menu")] -> w178
            frame False {
            }
            frame True {
            }
          }
          n122 = case shown="True" w187 {
            tunnel: [DIO_Update_Ops."get" ("menu") DIO_Update_Ops."set value" ("menu")] -> w182
            frame False {
            }
            frame True {
            }
          }
          n123 = call "DIFF_SIM_POSE.vi"("in Sim Pose"=w167, "WRITE"=TRUE) -> ()  [unwired: 9 in, 1 out]
          n124 = call <vilib>:"MathUtil_InputModulus.vi"("Maximum_Input"=180.0, "Minimum_Input"=-180.0, "Input"=w158) -> ("modulus"=→"Heading Deg":dbl)  [unwired: 8 in]
          n125 = Multiply(x=12.0, y=w163) -> (x*y=→"Left Wheel\nInch / Sec":dbl)
          n126 = Multiply(x=12.0, y=w160) -> (x*y=→"Right Wheel\nInch / Sec":dbl)
          n127 = call <vilib>:"DIO_PanelSim_Global.vi"("menu"=DIO_Update_Ops."get", "DIO Channel"=FPGA_DIOChannel."DIO 3") -> ("DIO new"=w196:T5)  [unwired: 12 in, 1 out]
          "DIO 3\nOut" <- w196
          n128 = call <vilib>:"DIO_PanelSim_Global.vi"("menu"=w182, "DIO Channel"=FPGA_DIOChannel."DIO 2", "Value Set"="Button\n    C") -> ("DIO new"=w179:T5)  [unwired: 11 in, 1 out]
          "DIO 2\nIn / Out" <- w179
          n129 = call <vilib>:"DIO_PanelSim_Global.vi"("menu"=w178, "DIO Channel"=FPGA_DIOChannel."DIO 1", "Value Set"="Button\n    B") -> ("DIO new"=w176:T5)  [unwired: 11 in, 1 out]
          "DIO 1\nIn / Out" <- w176
          n130 = call <vilib>:"DIO_PanelSim_Global.vi"("menu"=w175, "DIO Channel"=FPGA_DIOChannel."DIO 0", "Value Set"="Button\n    A") -> ("DIO new"=→"DIO 0\nIn":T5)  [unwired: 11 in, 1 out]
          n131 = Unbundle By Name(w176) -> ("data.<>value"=→"Green LED\nDIO 1":bool)
          n132 = Unbundle By Name(w179) -> ("data.<>value"=→"Red LED\nDIO 2":bool)
          n133 = Unbundle By Name(w196) -> ("data.<>value"=→"Yellow LED\nDIO 3":bool)
        }
      }
    }
  }
